vi "addActions.vi"(8 "Error In":errorcluster, 10 "actions":refnum<class "QAction.lvclass">[](array[class]), 11 "QWidget In":refnum<class "QWidget.lvclass">) -> (0 "Error Out":errorcluster, 3 "QWidget Out":refnum<class "QWidget.lvclass">)   [LabVIEW 2014, in "QWidget.lvclass"]
doc: "LabVIEW-specific documentation is not yet available. See <b>https://doc.qt.io/qt-5/qwidget.html#addActions</b>"
uses:
  QWidget.lvclass
  QAction/QAction.lvclass
  LQ Core/LQIdentity/LQIdentity.lvclass/LQIdentity.ctl
  LQ Core/LQ Core.lvlib
  LQ Core/LQIdentity/LQIdentity.lvclass
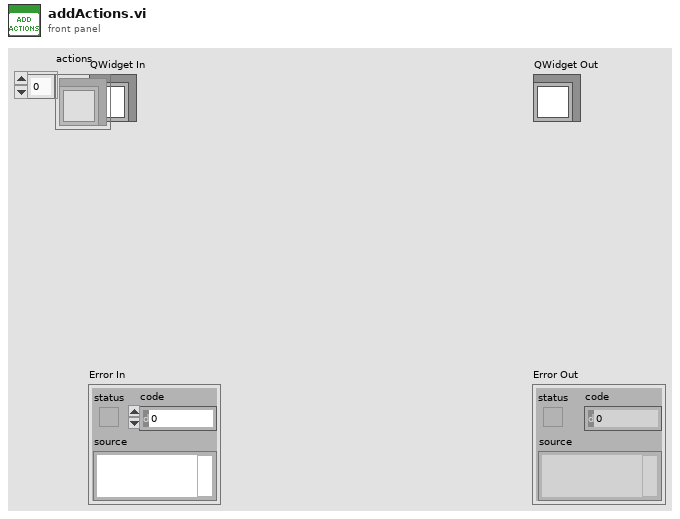
[diagram p1: front panel]
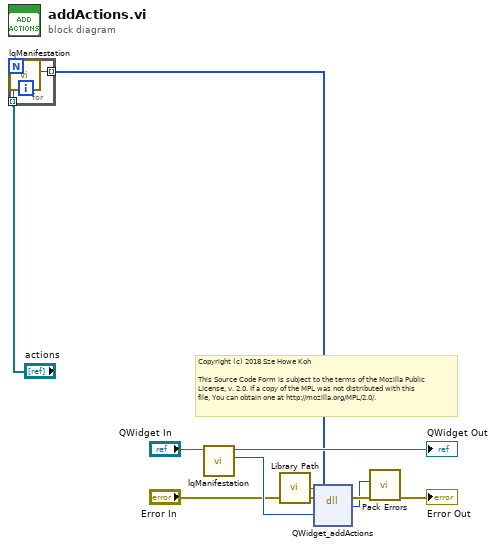
[diagram p0: block diagram]
diagram:
  # "Copyright (c) 2018 Sze Howe Koh\n\nThis Source Code Form is subject to the terms of the Mozilla Public\nLicense, v. 2.0. If a copy of the MPL was not distributed with this\nfile, You can obtain one at http://mozilla.org/MPL/2.0/."
  n1 = for {
    tunnel: "actions" -> [w12] mode=indexing
    tunnel: [w11] -> w1 mode=indexing
    n2 = call "lqManifestation.vi"("LQIdentity in"=w12) -> ("Manifestation"=w11:u64)  [unwired: 9 in, 1 out]
  }
  n3 = call "lqManifestation.vi"("LQIdentity in"="QWidget In") -> ("Manifestation"=w7:u64, "LQIdentity out"=→"QWidget Out":refnum<class "QWidget.lvclass">)  [unwired: 9 in]
  n4 = call "Library Path.vi"() -> ("Library Path"=w8:path)
  n5 = dll-call lib="?" fn="QWidget_addActions"(path in=w8, error in="Error In", "_instance"=w7, "actions"=w1) -> (error out=w5:errorcluster, w3:i32)  [unwired: 3 in, 1 out]
  n6 = call "Pack Errors.vi"("Error In"=w5, "Error Code"=w3) -> ("Error Out"=→"Error Out":errorcluster)  [unwired: 9 in]
